vi "read remote chassis.vi"(8 "error in":errorcluster, 11 "controller in":refnum<class "Controller.lvclass">) -> (0 "error out":errorcluster, 2 "remote chassis":refnum<class "Chassis.lvclass">[](array[class]), 3 "controller out":refnum<class "Controller.lvclass">)   [LabVIEW 2013, in "SMI.lvlib" / "Controller.lvclass"]
uses:
  Controller.lvclass
  Chassis/Chassis.lvclass
  Controller.lvclass/Controller.ctl
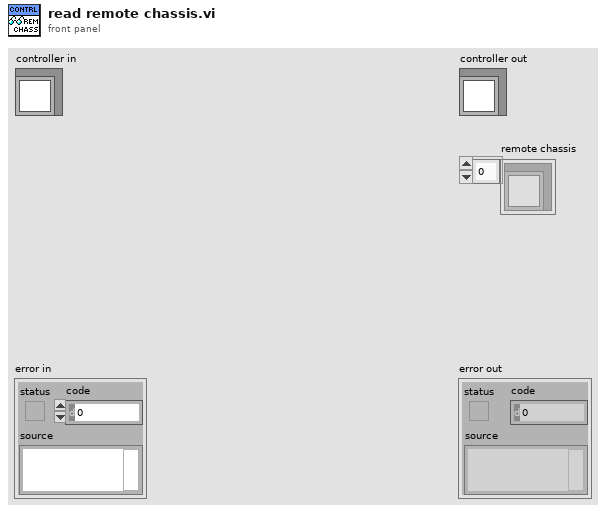
[diagram p1: front panel]
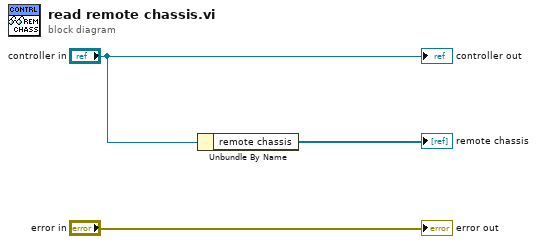
[diagram p0: block diagram]
diagram:
  n1 = Unbundle By Name("controller in") -> ("remote chassis"=→"remote chassis":refnum<class "Chassis.lvclass">[])
  "error out" <- "error in"
  "controller out" <- "controller in"
